vi "Append User Formatted HTML to Report.vi"(0 "report in":refnum<class "NI_HTML.lvclass">, 5 "HTML text":string, 11 "error in (no error)":errorcluster) -> (4 "report out":refnum<class "NI_HTML.lvclass">, 15 "error out":errorcluster)   [LabVIEW 2015, in "NI_HTML.lvclass"]
doc: "Inserts text that is not LabVIEW preformatted in the HTML report. You cannot use this VI with standard reports."
uses:
  <vilib>/Utility/NIReport.llb/HTML/NI_HTML.lvclass
  <vilib>/Utility/NIReport.llb/HTML/NI_HTML.lvclass/NI_HTML.ctl
  <vilib>/Utility/NIReport.llb/NI_ReportGenerationCore.lvlib
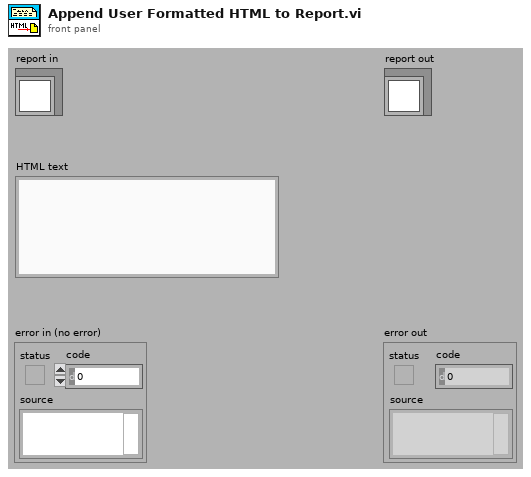
[diagram p1: front panel]
types:
  T1 = typedef "NI_ReportGenerationCore.lvlib/HTML Report Data.ctl" = cluster{"Body Text":string, "Font Tag":string, "Title Text":string, "Header Text":string, "Footer Text":string, "Image List":path[]}
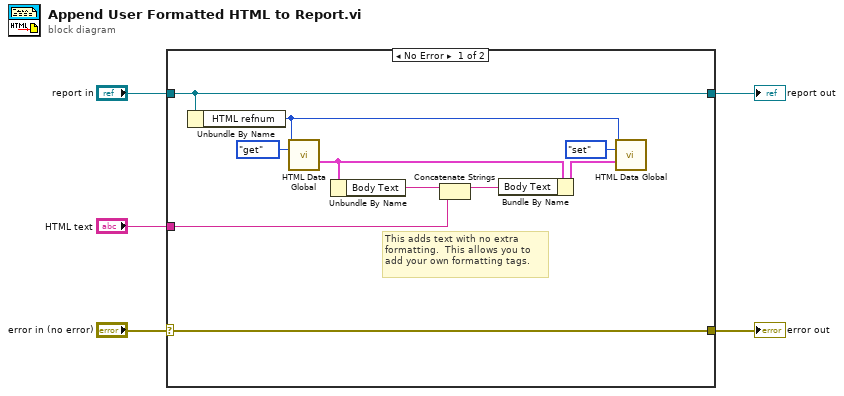
[diagram p0: block diagram]
diagram:
  n1 = case shown="No Error" "error in (no error)" {
    selector: "error in (no error)" -> [w15 w17]
    tunnel: [w15 w17] -> w4
    tunnel: [w10 w16] -> w2
    tunnel: "report in" -> [w10 w16]
    tunnel: "HTML text" -> [w12 _]
    frame No Error {
      # "This adds text with no extra \nformatting.  This allows you to \nadd your own formatting tags."
      n2 = Unbundle By Name(w10) -> ("HTML refnum"=w6:u32)
      n3 = call <vilib>:"HTML Data Global.vi"("HTML refnum"=w6, "menu"=enum16{"init", "get", "set", "delete"}."get") -> ("HTML report data out"=w7:T1)  [unwired: 1 in, 12 out]
      n4 = Unbundle By Name(w7) -> ("Body Text"=w14:string)
      n5 = Concatenate Strings(w14, w12) -> (w13:string)
      n6 = Bundle By Name(cluster=w7, "Body Text"=w13) -> (w8:T1)
      n7 = call <vilib>:"HTML Data Global.vi"("HTML refnum"=w6, "menu"=enum16{"init", "get", "set", "delete"}."set", "HTML report data in"=w8) -> ()  [unwired: 13 out]
    }
    frame Error {
    }
  }
  "error out" <- w4
  "report out" <- w2
